vi "Configure Power On State.vi"(7 "Slave Address":i32=-1 min=-1 max=30 step=1, 8 "error":errorcluster, 10 "Power-On":enum16{"Safe-Start", "Auto-Start"}(ring), 11 "VISA":refnum<visa-resource-name>) -> (0 "error out":errorcluster, 3 "VISA out":refnum<visa-resource-name>)   [LabVIEW 2025, in "TDK-Lambda GEN LAN Series.lvlib"]
doc: "Configure the Power-On state of the power supply. The output enumerated type may be:\n\n(0) Safe Start. The power-supply will power-up with its output is off. Also, after any fault is cleared, the output will remain off.\n(1) Auto-Start. The power-supply will power-up in it's last state before the power was turned off. Also, after a non-latching faults is cleared, the output will turn back on automatically."
uses:
  <userlib>/TDK-Lambda GEN LAN Series/TDK-Lambda GEN LAN Series.lvlib
panel:
  # "Set Power-On State,\nSafe-Start or Auto-Start"
  # "TDK-Lambda Genesys \n LAN\n  DC Power Supplies"
  # "(c) 2019 TDK-Lambda.  ALL RIGHTS RESERVED."
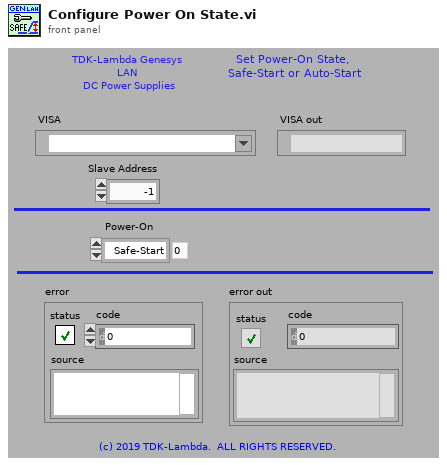
[diagram p1: front panel]
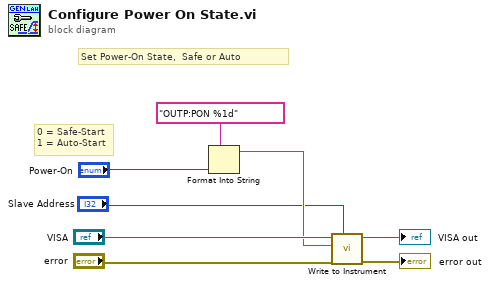
[diagram p0: block diagram]
diagram:
  # "0 = Safe-Start\n1 = Auto-Start"
  # "Set Power-On State,  Safe or Auto"
  n1 = Format Into String(format string="OUTP:PON %1d", "Power-On") -> (resulting string=w2:string)  [unwired: 2 in, 1 out]
  n2 = call <userlib>:"Write to Instrument.vi"("Slave Address"="Slave Address", "error"="error", "Command"=w2, "VISA"="VISA") -> ("error out"=→"error out":errorcluster, "VISA out"=→"VISA out":refnum<visa-resource-name>)  [unwired: 6 in]
